vi "Get Tool Analog Vars.vi"(11 "error in (no error)":errorcluster) -> (4 "Catagorised  Stsaus":T1[](array[typedef]), 6 "Values":dbl[](array[numeric]), 8 "Analog Vars":T4[](array[typedef]) {"Value" format="%#.1f"}, 10 "Alarm":bool, 13 "Action":T3 items=["No Action", "Turn Off HV"], 14 "Alarms":bool[](array[boolean]), 15 "error out":errorcluster)   [LabVIEW 2011]
uses:
  GUI/Analog Var Disp 0 sif.ctl
  GUI/Status indicator Black Small.ctl
  Measurments Handling/Action List.ctl
  Measurments Handling/Catagorised alarm state.ctl
  GUI/Status Indikator Helper.ctl
  Measurments Handling/Action Analog Handler.ctl
  Measurments Handling/Common/Variable List Common Analog.ctl
  <vilib>/Utility/VariantDataType/GetNumericInfo.vi
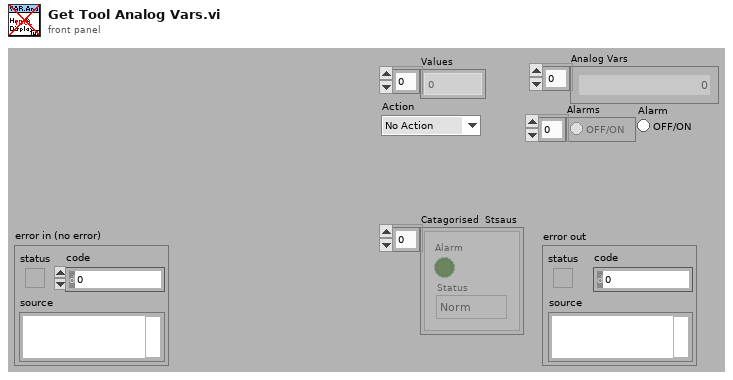
[diagram p1: front panel]
types:
  T1 = typedef "Catagorised alarm state.ctl" = cluster{"Alarm":bool, "Status":T2}
  T2 = typedef "Status Indikator Helper.ctl" = enum16{"Norm", "L", "H", "LL", "HH", "Value", "Technical"}
  T3 = typedef "Action List.ctl" = u16
  T4 = typedef "Analog Var Disp 0 sif.ctl" = cluster{"Value":dbl, "Unit":string, "Status":T5}
  T5 = typedef "Status indicator Black Small.ctl" = u16
  T6 = typedef "Variable List Common Analog.ctl" = enum16{"HVPSU Head Voltage", "HVPSU TS Voltage", "HVPSU Current", "PCP Cable Resistance", "Winch Depth", "Winch Line Speed", "Winch Wire Tension"}
  T7 = typedef "Action Analog Handler.ctl" = enum16{"GET value", "GET Single Frequenzy", "GET All Values", "GET Waveform", "Get Numb Var", "SET Value", "START Buffer", "REG Variable", "BUF size(total antal sekund)", "PULS", "Get a Value at time", "Set initial waveform"}
  T8 = typedef "User Setting Analog Channel Bg.ctl" = cluster{"Scaling":T9, "Limits and responces":T10, "Allow Graph selection by user":bool, "Unit":u16}
  T9 = typedef "Scaling.ctl" = cluster{"Gain":dbl, "Offset":dbl}
  T10 = typedef "Alarm Setup Analog.ctl" = cluster{"Technical Error(NA)":T11, "LL":T11, "L":T11, "H":T11, "HH":T11, "Limits":T12}
  T11 = typedef "Alarm Responce.ctl" = cluster{"Action":T3, "Alarm":bool}
  T12 = typedef "Limits.ctl" = cluster{"LL":dbl, "L":dbl, "H":dbl, "HH":dbl}
  T13 = typedef "Fixed Analog Channel Definition.ctl" = cluster{"ID":u16, "Name":string, "Quantity":T14, "Unit":string, "Maximum upd":T15, "Comment":string, "Help file Name":string, "Help file Section ":string, "Category":T16, "User adjustable Scaling":bool, "Default Scaling":T9, "In use":bool, "Default Unit":i32}
  T14 = typedef "Quantity enum.ctl" = enum16{"Acceleration", "Angle", "Current", "Force", "Distance", "Pressure", "Resistance", "Rotational Speed", "Speed", "Temperature", "Tension", "Torque", "Voltage", "Weight"}
  T15 = typedef "Update frequensies.ctl" = enum16{"2 Hz", "1 Hz", "0.1 Hz"}
  T16 = typedef "Channel catagory Enum.ctl" = enum16{"No Category", "Power", "Temperature", "Pressure"}
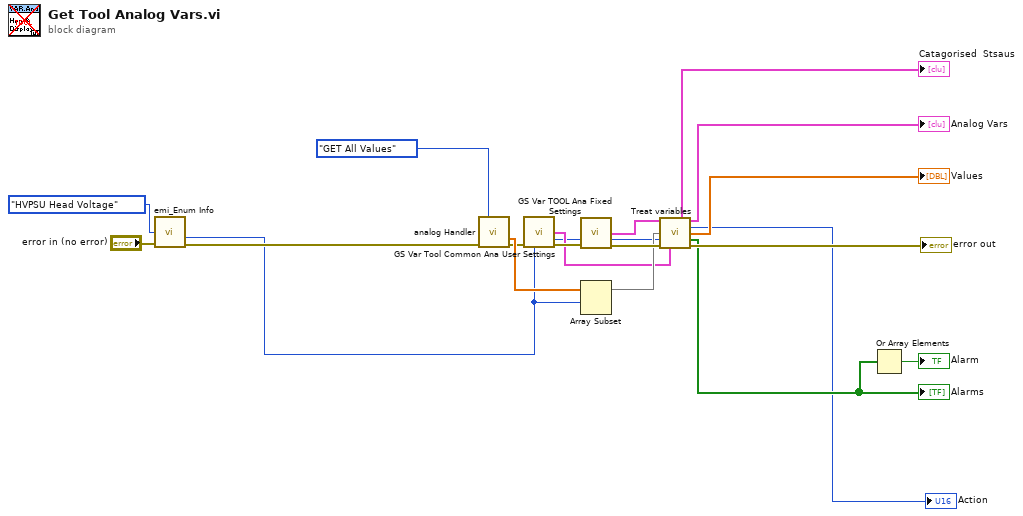
[diagram p0: block diagram]
diagram:
  n1 = call "emi_Enum Info.vi"("Enum"=Variable_List_Common_Analog."HVPSU Head Voltage" ("Action"), "error in (no error)"="error in (no error)") -> ("Numb Elements"=w2:i32, "error out"=w14:errorcluster)  [unwired: 10 in, 2 out]
  n2 = call "analog Handler.vi"("Action"=Action_Analog_Handler."GET All Values" ("Action(GET)"), "error in (no error)"=w14) -> ("Values"=w19:dbl[], "error out"=w13:errorcluster)  [unwired: 8 in, 4 out]
  n3 = call "GS Var Tool Common Ana User Settings.vi"("error in (no error)"=w13) -> ("Tool Analog var User settigns out"=w8:T8[], "error out"=w12:errorcluster)  [unwired: 12 in, 1 out]
  n4 = call "GS Var TOOL Ana Fixed Settings.vi"("error in (no error)"=w12) -> ("Tool Analog var Fixed out"=w10:T13[], "error out"=w11:errorcluster)  [unwired: 12 in, 1 out]
  n5 = Array Subset(array=w19, index=w2) -> (w9:dbl[])  [unwired: 1 in]
  n6 = call "Treat variables.vi"("Analog Variable info fixed"=w10, "Analog values"=w9, "Variabel start index"=w2, "error In"=w11, "Analog Variable info Settings"=w8) -> ("Catagorised  Stsaus"=→"Catagorised  Stsaus":T1[], "Analog Variable Display"=→"Analog Vars":T4[], "Action"=→"Action":T3, "Analog Values"=→"Values":dbl[], "Alarms"=w4:bool[], "error out"=→"error out":errorcluster)  [unwired: 5 in]
  "Alarms" <- w4
  n7 = Or Array Elements(Boolean array=w4) -> (logical OR=→"Alarm":bool)
